vi "Pre-Uninstall Custom Action.vi"(10 "Variant":variant) -> (0 "error out":errorcluster)   [LabVIEW 2017]
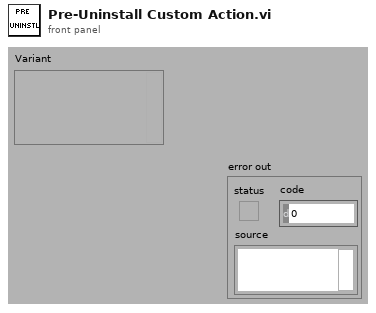
[diagram p1: front panel]
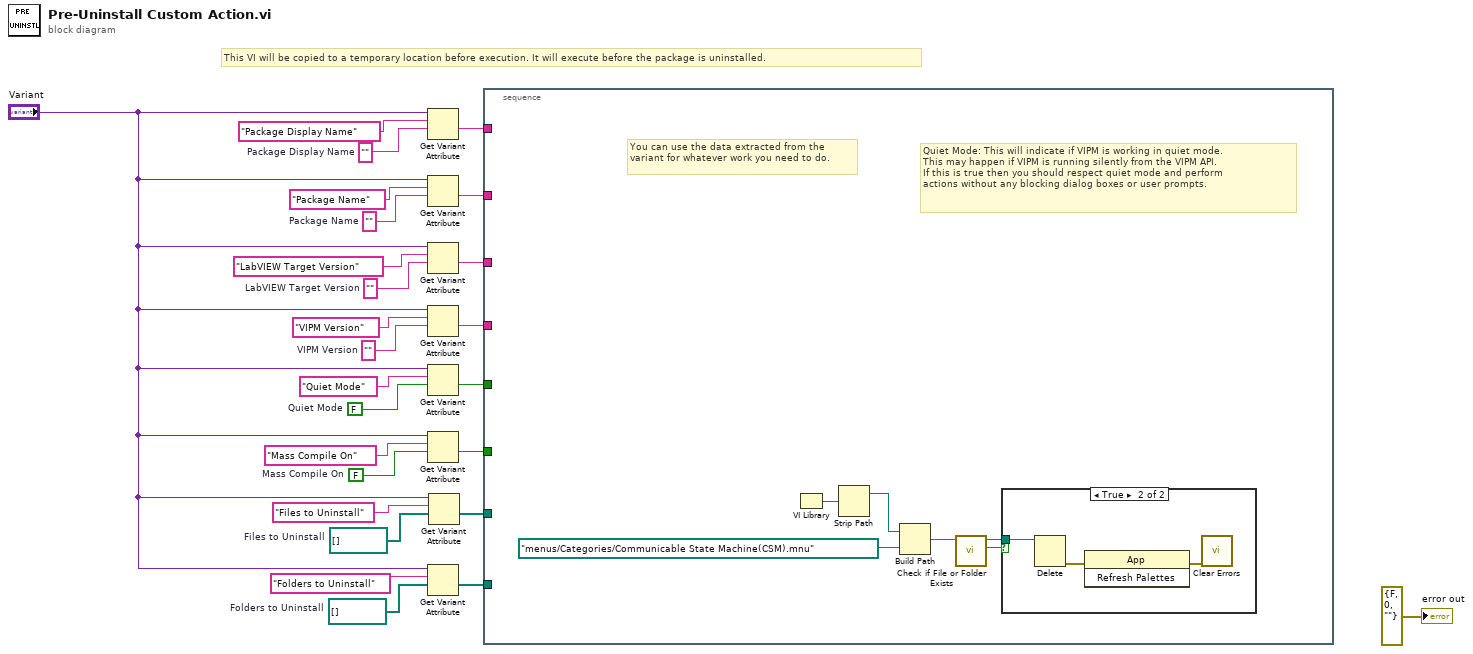
[diagram p0: block diagram]
diagram:
  w3 = path[] []  # Folders to Uninstall
  w7 = path[] []  # Files to Uninstall
  w8 = FALSE  # Mass Compile On
  w9 = ""  # Package Display Name
  w16 = FALSE  # Quiet Mode
  w19 = ""  # VIPM Version
  w21 = ""  # LabVIEW Target Version
  w23 = ""  # Package Name
  # "This VI will be copied to a temporary location before execution. It will execute before the package is uninstalled."
  n1 = Get Variant Attribute(Variant="Variant", name="Package Display Name", default value (empty Variant)=w9) -> (value=w15:string)  [unwired: 1 in, 3 out]
  n2 = Get Variant Attribute(Variant="Variant", name="Package Name", default value (empty Variant)=w23) -> (value=w14:string)  [unwired: 1 in, 3 out]
  n3 = Get Variant Attribute(Variant="Variant", name="LabVIEW Target Version", default value (empty Variant)=w21) -> (value=w13:string)  [unwired: 1 in, 3 out]
  n4 = Get Variant Attribute(Variant="Variant", name="VIPM Version", default value (empty Variant)=w19) -> (value=w12:string)  [unwired: 1 in, 3 out]
  n5 = Get Variant Attribute(Variant="Variant", name="Quiet Mode", default value (empty Variant)=w16) -> (value=w11:bool)  [unwired: 1 in, 3 out]
  n6 = Get Variant Attribute(Variant="Variant", name="Mass Compile On", default value (empty Variant)=w8) -> (value=w10:bool)  [unwired: 1 in, 3 out]
  n7 = Get Variant Attribute(Variant="Variant", name="Folders to Uninstall", default value (empty Variant)=w3) -> (value=w2:path[])  [unwired: 1 in, 3 out]
  n8 = Get Variant Attribute(Variant="Variant", name="Files to Uninstall", default value (empty Variant)=w7) -> (value=w5:path[])  [unwired: 1 in, 3 out]
  n9 = stacked-sequence {
    tunnel: w15 -> [_]
    tunnel: w14 -> [_]
    tunnel: w13 -> [_]
    tunnel: w12 -> [_]
    tunnel: w11 -> [_]
    tunnel: w10 -> [_]
    tunnel: w5 -> [_]
    tunnel: w2 -> [_]
    frame #0 {
      # "Quiet Mode: This will indicate if VIPM is working in quiet mode.\nThis may happen if VIPM is running silently from the VIPM API.\nIf this is true then you should respect quiet mode and perform\nactions without any blocking dialog boxes or user prompts."
      # "You can use the data extracted from the variant for whatever work you need to do."
      n10 = VI Library() -> (path=w28:path)
      n11 = Strip Path(path=w28) -> (stripped path=w27:path)  [unwired: 1 out]
      n12 = Build Path(base path=w27, name or relative path=path "menus/Categories/Communicable State Machine(CSM).mnu") -> (appended path=w31:path)
      n13 = call <vilib>:"Check if File or Folder Exists.vi"("path"=w31) -> ("file or folder exists?"=w29:bool, "dup path"=w30:path)  [unwired: 8 in, 1 out]
      n14 = case shown="True" w29 {
        tunnel: w30 -> [_ w34]
        frame False {
        }
        frame True {
          n15 = Delete(path (use dialog)=w34) -> (error out=w35:errorcluster)  [unwired: 4 in, 2 out]
          n16 = invoke class="App" method="Refresh Palettes"(error in=w35) -> (error out=w33:errorcluster)  [unwired: 2 in, 2 out]
          n17 = call <vilib>:"Clear Errors.vi"("error in (no error)"=w33) -> ()  [unwired: 5 in, 2 out]
        }
      }
    }
  }
  "error out" <- errorcluster {"status"=FALSE, "code"=0, "source"=""} ("error out")
